vi "Configure Serial Input Power Over Coax Source.vi"(0 "fpga interface in":refnum<k20>, 5 "serial input channels":string[](array[string]), 7 "power over coax source":i32(ring) items=["None", "Internal", "Auxiliary"], 9 "power over coax in range timeout (s)":dbl=5.0, 11 "error in (no error)":errorcluster) -> (4 "fpga interface out":refnum<k20>, 6 "power over coax source in range":bool[](array[boolean]), 15 "error out":errorcluster)   [LabVIEW 2023, in "GettingStarted_Common_148X_Host.lvlib"]
uses:
  GettingStarted_Common_148X_Host.lvlib
  <instrlib>/FlexRIO/API/Host/v1/NI FlexRIO/API/Get Property Reference - Fpga Small.vi
  <resource>/objmgr/niflexrioapiChannel.rc
  <instrlib>/FlexRIO/API/Host/v1/NI FlexRIO API v1.lvlib
  <resource>/objmgr/niflexrioapi.rc
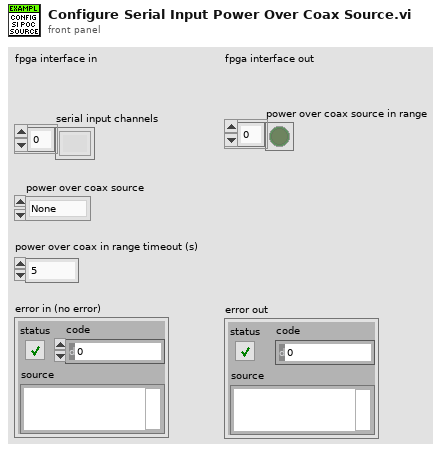
[diagram p1: front panel]
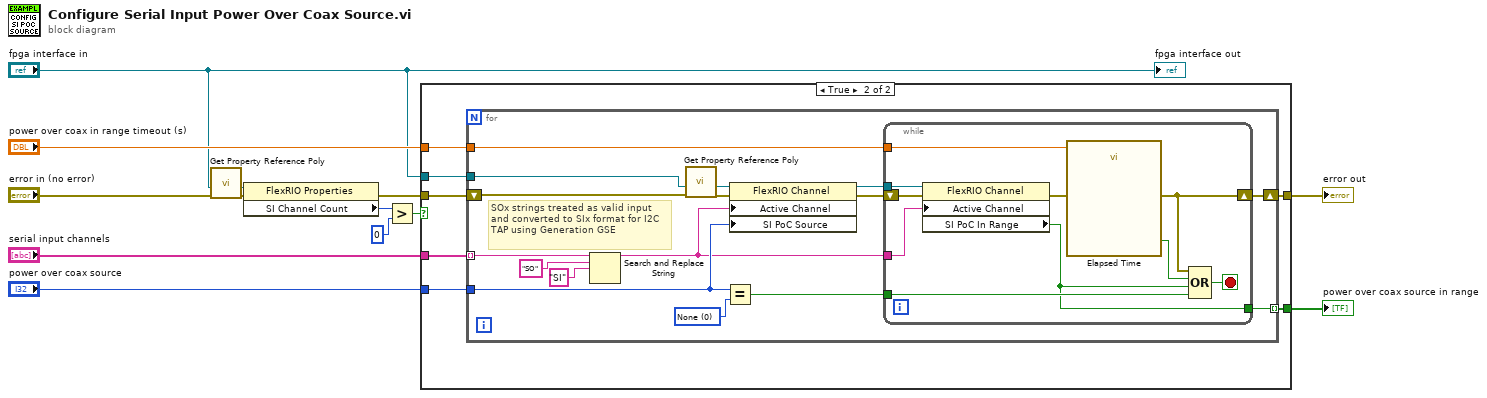
[diagram p0: block diagram]
diagram:
  n1 = call-poly <instrlib>:"Get Property Reference Poly.vi"("error in (no error)"="error in (no error)", "fpga interface in"="fpga interface in") -> ("error out"=w7:errorcluster, "property reference"=w8:refnum<k20>)  [unwired: 4 in, 1 out]
  n2 = property class="FlexRIO Properties"(reference=w8, error in=w7) -> (error out=w2:errorcluster, "SI Channel Count"=w6:i32)  [unwired: 1 out]
  n3 = Greater?(x=w6, y=0) -> (0:w1:bool)
  n4 = case shown="True" w1 {
    tunnel: w2 -> [w14 w21]
    tunnel: "serial input channels" -> [_ w20]
    tunnel: [w14 w19] -> w12
    tunnel: "fpga interface in" -> [_ w18]
    tunnel: "power over coax source" -> [_ w17]
    tunnel: "power over coax in range timeout (s)" -> [_ w16]
    tunnel: [_ w15] -> w9
    frame False {
    }
    frame True {
      n5 = for {
        tunnel: w18 -> [w37]
        tunnel: w20 -> [w25] mode=indexing
        shift-right: [w34] -> w19
        shift-left: w21 -> [w22]
        tunnel: w17 -> [w31]
        tunnel: w16 -> [w29]
        tunnel: [w28] -> w15 mode=indexing
        w32 = 0 items=["None", "Internal", "Auxiliary"] ("Serial Input Power Over Coax Source 2")
        # "SOx strings treated as valid input and converted to SIx format for I2C TAP using Generation GSE"
        n6 = Search and Replace String(input string=w25, search string="SO", replace string="SI" ("replace string (\"\")")) -> (result string=w24:string)  [unwired: 5 in, 3 out]
        n7 = call-poly <instrlib>:"Get Property Reference Poly.vi"("error in (no error)"=w22, "fpga interface in"=w37) -> ("error out"=w23:errorcluster, "property reference"=w30:refnum<k20>)  [unwired: 4 in, 1 out]
        n8 = Equal?(x=w31, y=w32) -> (x = y?=w33:bool)
        n9 = property class="FlexRIO Channel"(reference=w30, error in=w23, "Active Channel"=w24, "SI PoC Source"=w31) -> (reference out=w36:refnum<k20>, error out=w35:errorcluster)
        n10 = while {
          tunnel: w36 -> [w46]
          tunnel: w24 -> [w45]
          tunnel: w33 -> [w43]
          shift-right: [w38] -> w34
          shift-left: w35 -> [w47]
          tunnel: w29 -> [w40]
          tunnel: [w39] -> w28
          stop <- w44 stop-if-true
          n11 = property class="FlexRIO Channel"(reference=w46, error in=w47, "Active Channel"=w45) -> (error out=w42:errorcluster, "SI PoC In Range"=w39:bool)  [unwired: 1 out]
          n12 = call "Elapsed Time"("Time Target (s)"=w40, "error in (no error)"=w42) -> ("Time has Elapsed"=w41:bool, "error out"=w38:errorcluster)  [unwired: 10 in, 6 out]
          n13 = Compound Arithmetic op=OR(w38, w41, w39, w43) -> (w44:bool)
        }
      }
    }
  }
  "error out" <- w12
  "power over coax source in range" <- w9
  "fpga interface out" <- "fpga interface in"
